vi "Find Resonances ASPT.vi"(8 "Error In":errorcluster, 11 "File Path Control":path=path "C:/Data/Spectra for Fedor/Ok spectra/300.00000K_175_555_2.10000V_0.00000T_May20-2015__09-37-18_001_052015.tdms") -> (0 "Error Out":errorcluster)   [LabVIEW 2016]
uses:
  Measure_extentions/Post-Processors/Line Detector/Line Detector Configuration.ctl
  <vilib>/Analysis/3filter.llb/Filter Passband Type.ctl
  <vilib>/Analysis/3filter.llb/Bessel Filter (CDB).vi
  Smooth Background CDBL.vi
  <vilib>/addons/Wavelet Analysis/application.llb/WA Multiscale Peak Detection (Array).vi
  <vilib>/Analysis/NI_AALPro.lvlib
  <vilib>/Analysis/NI_AAL_SigProc.lvlib
  <vilib>/Analysis/NI_AALBase.lvlib
  <vilib>/addons/_Advanced Signal Processing/NI_AdvSigProcWA.lvlib
panel:
  in  "ASPT?":bool
  out "# found":i32
  out "error":i32
  in  "Low pass distortion":dbl
  out "XY Graph 6":cluster{dbl[], dbl[]}[](graph)
  in  "User configuration":T1={"Peak width"=30.0} {"Peak width" format="%#_6pHz"}
  in  "Signal channel":string="Signal"
  in  "Frequency channel":string="Frequency"
  in  "group name in":string="p"
  in  "HP F":dbl=0.1 format="%#_6p"
  in  "LP  F":dbl=0.001 format="%#_6p"
  in  "Fit?":bool
  in  "Complex":bool
  in  "Deviations":dbl=1.0
  out "variance":dbl format="%.2p"
  out "standard deviation":dbl format="%.2p"
  out "Peak F":dbl format="%#_6pHz"
  in  "Points around peak":i32=100
  in  "Peak number":i32
  out "XY Graph 5":cluster{"Array":dbl[], "Array":dbl[]}[](graph)
  out "width":i32=100 min=3
  out "XY Graph 4":cluster{"Y":dbl[], dbl[]}(graph)
  out "XY Graph 3":cluster{"Y":dbl[], "Y":dbl[]}[](graph)
  out "Magnitude":cluster{"Y":dbl[], dbl[]}[](graph)
  out "Phase":cluster{"Y":dbl[], "Unwrapped Phase":dbl[]}[](graph)
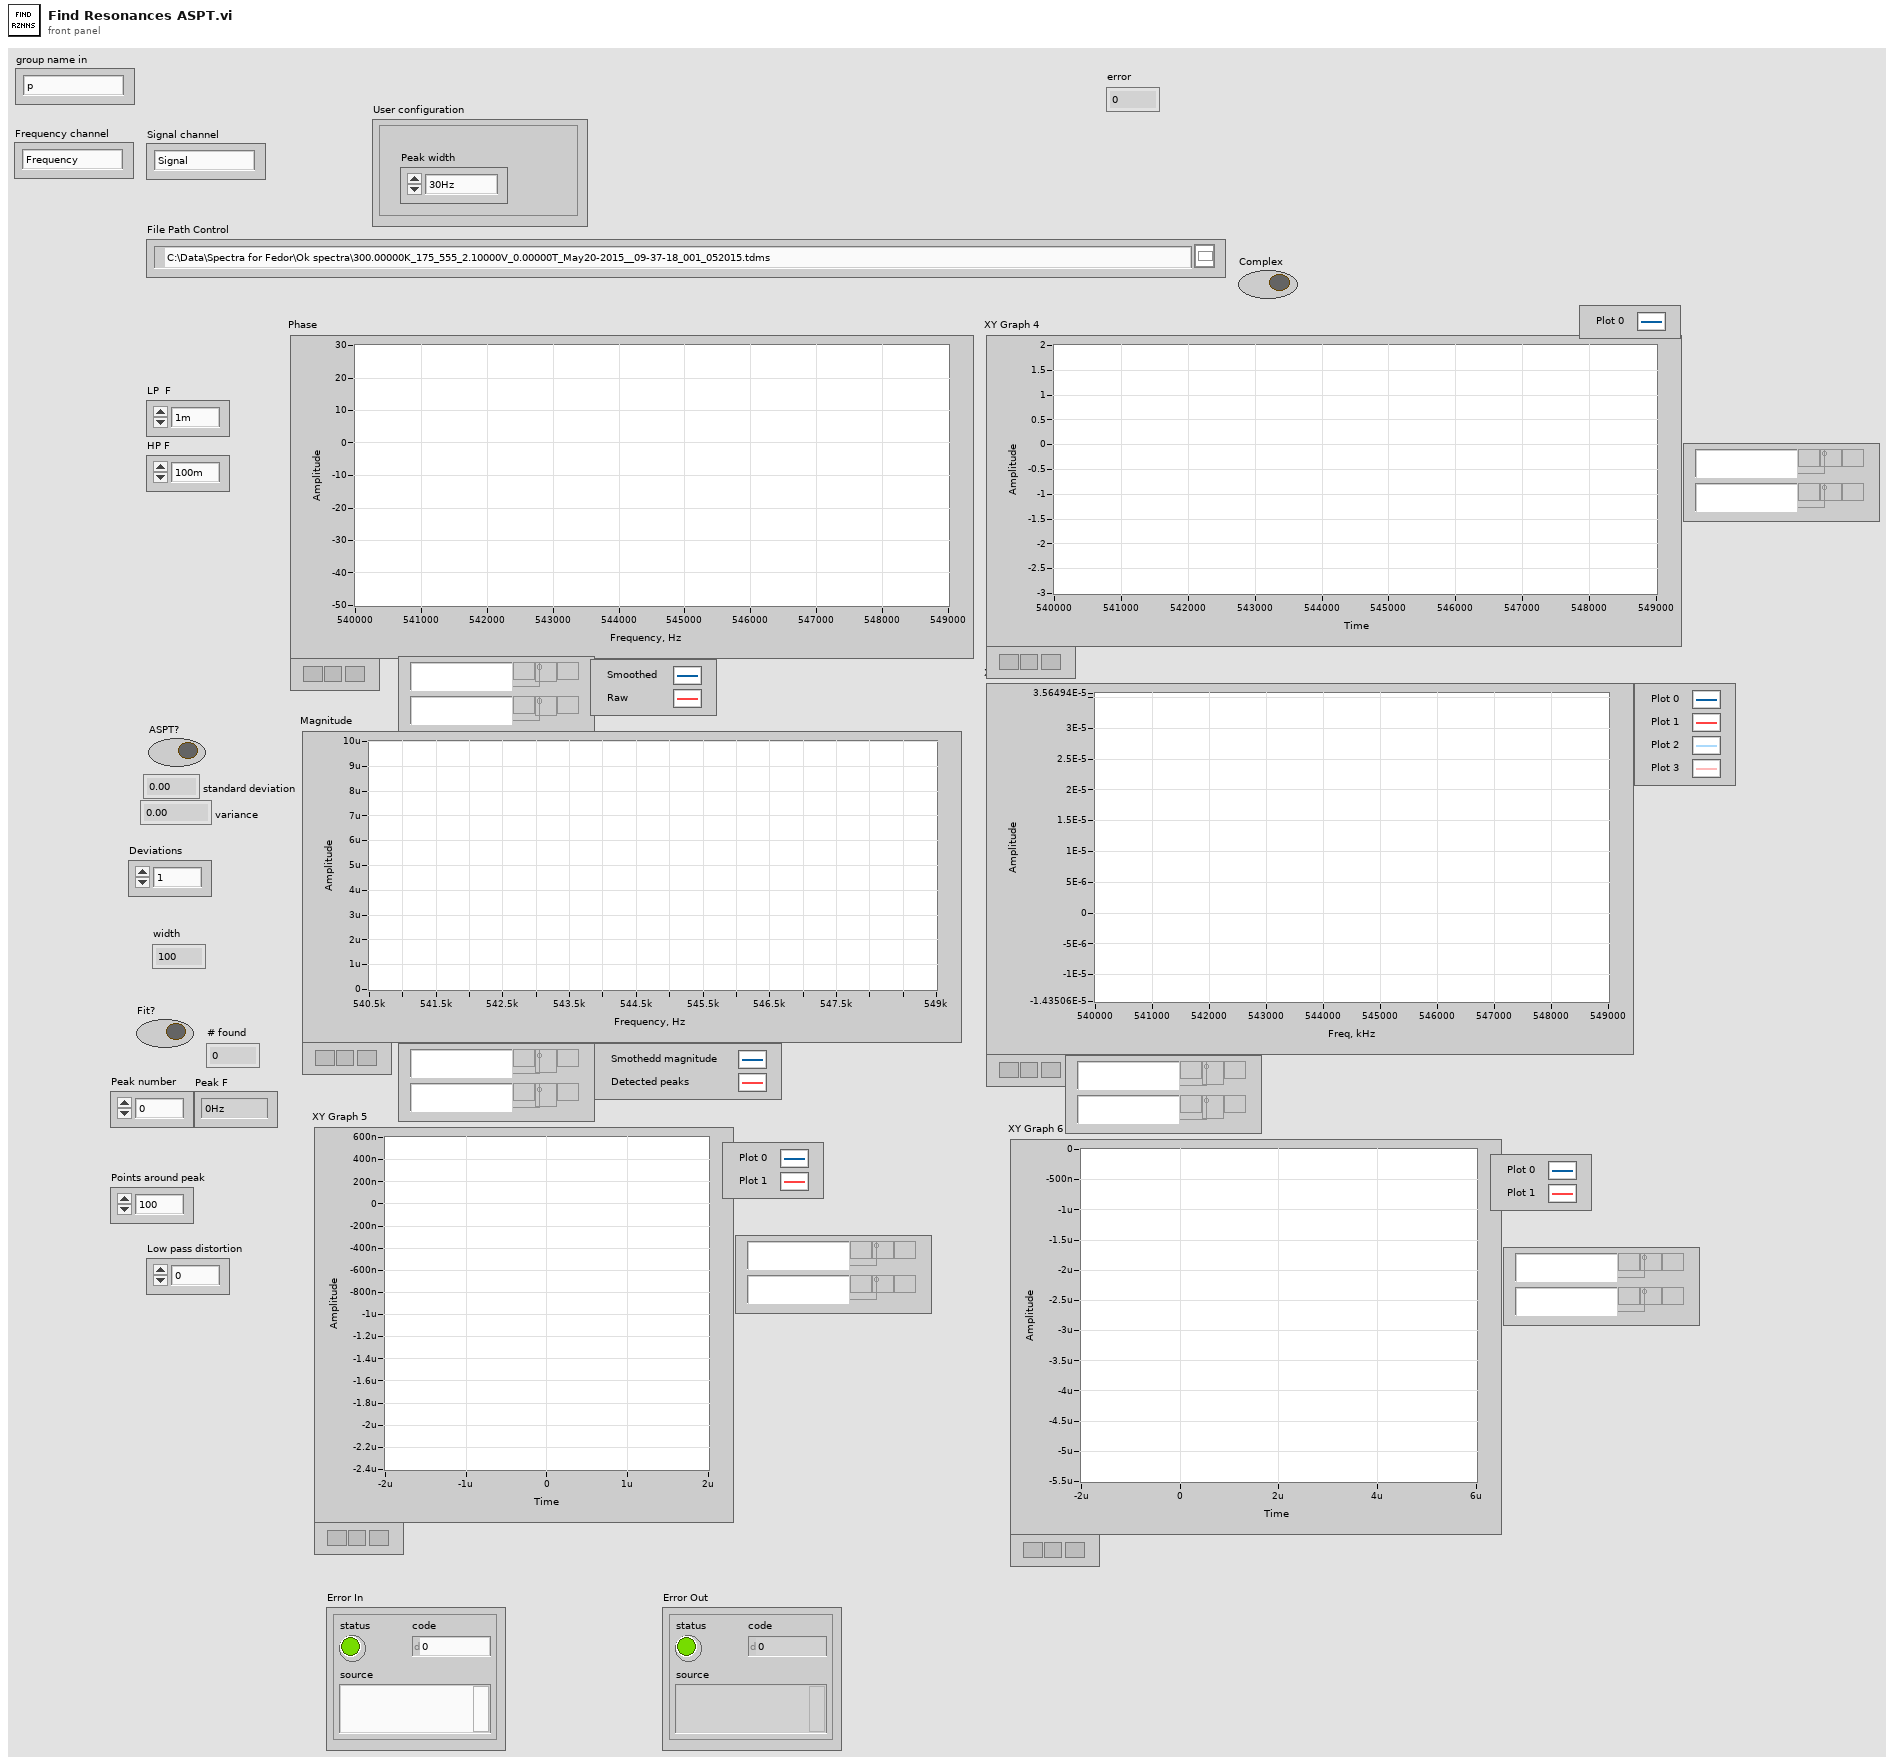
[diagram p1: front panel]
types:
  T1 = typedef "Line Detector Configuration.ctl" = cluster{"Peak width":dbl}
  T2 = enum16{"open", "open or create", "create or replace", "create", "open (read-only)"}
  T3 = typedef "NI_AALBase.lvlib/Filter Passband Type.ctl" = enum32{"Lowpass", "Highpass", "Bandpass", "Bandstop"}
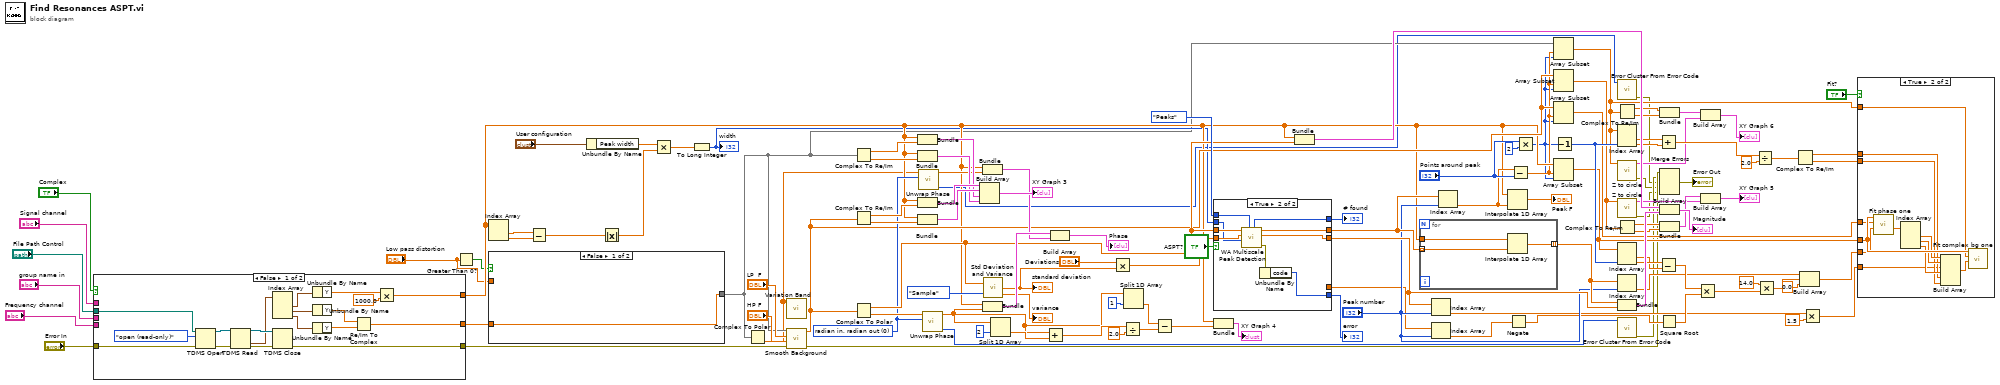
[diagram p0: block diagram]
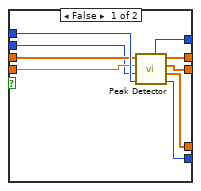
[diagram p2: hidden frame]
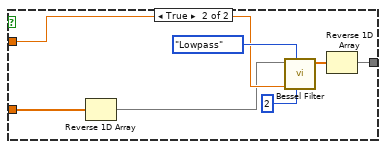
[diagram p3: hidden frame]
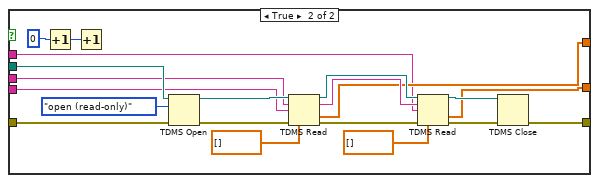
[diagram p5: hidden frame]
diagram:
  w81 = 0 items=["radian in, radian out", "radian in, degree out", "degree in, degree out", "degree in, radian out"] ("phase unit")
  n1 = case shown="False" "Complex" {
    tunnel: "File Path Control" -> [w137 w157]
    tunnel: [w121 w141] -> w40
    tunnel: "group name in" -> [_ w146]
    tunnel: "Frequency channel" -> [_ w145]
    tunnel: [w124 w142] -> w14
    tunnel: "Signal channel" -> [_ w140]
    tunnel: "Error In" -> [w123 w139]
    tunnel: [w122 w138] -> w41
    frame False {
      n2 = TDMS Open(8:w123, 10:T2."open (read-only)" ("operation (0:open)"), 11:w137) -> (0:w134:errorcluster, 3:w135:refnum<k34>)  [unwired: 4 in]
      n3 = TDMS Read(0:w135, 11:w134) -> (4:w133:refnum<k34>, 10:w131:waveform(dbl)[], 15:w132:errorcluster)  [unwired: 6 in, 3 out]
      n4 = Index Array(array=w131) -> (element #1=w130:waveform(dbl), element #2=w128:waveform(dbl), element #3=w129:waveform(dbl))  [unwired: 3 in]
      n5 = TDMS Close(8:w132, 11:w133) -> (0:w122:errorcluster)  [unwired: 1 out]
      n6 = Unbundle By Name(w130) -> ("Y"=w127:dbl[])
      n7 = Unbundle By Name(w128) -> ("Y"=w126:dbl[])
      n8 = Unbundle By Name(w129) -> ("Y"=w125:dbl[])
      n9 = Re/Im To Complex(1:w125, 2:w126) -> (0:w124:cdb[])
      n10 = Multiply(x=w127, y=1000.0) -> (x*y=w121:dbl[])
    }
    frame True {
      n11 = Increment(x=0 ("index")) -> (x+1=w151:i32)
      n12 = Increment(x=w151) -> ()  [unwired: 1 out]
      n13 = TDMS Open(8:w139, 10:T2."open (read-only)" ("operation (0:open)"), 11:w157) -> (0:w154:errorcluster, 3:w155:refnum<k34>)  [unwired: 4 in]
      n14 = TDMS Read(0:w155, 5:w146, 7:w145, 11:w154, 12:dbl[] []) -> (4:w149:refnum<k34>, 6:w147:string, 10:w141:dbl[], 15:w153:errorcluster)  [unwired: 3 in, 2 out]
      n15 = TDMS Read(0:w149, 5:w147, 7:w140, 11:w153, 12:cdb[] []) -> (4:w148:refnum<k34>, 10:w142:cdb[], 15:w150:errorcluster)  [unwired: 3 in, 3 out]
      n16 = TDMS Close(8:w150, 11:w148) -> (0:w138:errorcluster)  [unwired: 1 out]
    }
  }
  n17 = Greater Than 0?(x="Low pass distortion") -> (x > 0?=w16:bool)
  n18 = Index Array(array=w40) -> (element #1=w39:dbl, element #2=w38:dbl)  [unwired: 2 in]
  n19 = case shown="False" w16 {
    tunnel: w14 -> [w158 w165]
    tunnel: [w158 w159] -> w13
    tunnel: "Low pass distortion" -> [_ w162]
    frame False {
    }
    frame True {
      n20 = Reverse 1D Array(array=w165) -> (reversed array=w160:cdb[])
      n21 = call-poly <vilib>:"Bessel Filter.vi"("order"=2, "filter type"=Filter_Passband_Type."Lowpass", "low cutoff freq: fl"=w162, "X"=w160) -> ("Filtered X"=w164:cdb[])  [unwired: 4 in, 1 out]
      n22 = Reverse 1D Array(array=w164) -> (reversed array=w159:cdb[])
    }
  }
  n23 = Subtract(x=w39, y=w38) -> (x-y=w37:dbl)
  n24 = Unbundle By Name("User configuration") -> ("Peak width"=w35:dbl)
  n25 = Absolute Value(x=w37) -> (abs(x)=w34:dbl)
  n26 = Multiply(x=w35, y=w34) -> (x*y=w33:dbl)
  n27 = To Long Integer(number=w33) -> (32bit integer=w32:i32)
  "width" <- w32
  n28 = Complex To Polar(r * e^(i*theta)=w13) -> (theta=w2:dbl[])  [unwired: 1 out]
  n29 = call "Variation Band.vi"("Data"=w2) -> ()  [unwired: 11 in]
  n30 = call-poly "Smooth Background.vi"("Error In"=w41, "HP F"="HP F", "LP  F"="LP  F", "Data"=w13) -> ("Error Out"=w12:errorcluster, "Data out"=w52:cdb[])  [unwired: 6 in]
  n31 = Complex To Re/Im(x + iy=w13) -> (x=w91:dbl[], y=w92:dbl[])
  n32 = Complex To Re/Im(x + iy=w52) -> (x=w103:dbl[], y=w102:dbl[])
  n33 = Complex To Polar(r * e^(i*theta)=w52) -> (r=w88:dbl[], theta=w109:dbl[])
  n34 = Bundle(w40, w91) -> (w90:cluster{dbl[], dbl[]})  [unwired: 1 in]
  n35 = Bundle(w40, w92) -> (w89:cluster{dbl[], dbl[]})  [unwired: 1 in]
  n36 = Bundle(w40, w103) -> (w117:cluster{dbl[], dbl[]})  [unwired: 1 in]
  n37 = Bundle(w40, w102) -> (w116:cluster{dbl[], dbl[]})  [unwired: 1 in]
  n38 = call <vilib>:"Unwrap Phase.vi"("phase unit"=w81, "Phase"=w2) -> ("error"=w10:i32, "Unwrapped Phase"=w80:dbl[])  [unwired: 8 in]
  n39 = call <vilib>:"Unwrap Phase.vi"("phase unit"=w81, "Phase"=w109) -> ("error"=w11:i32, "Unwrapped Phase"=w104:dbl[])  [unwired: 8 in]
  n40 = Build Array(w117, w116, w90, w89) -> (→"XY Graph 3":cluster{dbl[], dbl[]}[])
  n41 = Bundle(w40, "Unwrapped Phase"=w80) -> (w78:cluster{dbl[], "Unwrapped Phase":dbl[]})  [unwired: 1 in]
  n42 = Bundle(w40, "Unwrapped Phase"=w104) -> (w118:cluster{dbl[], "Unwrapped Phase":dbl[]})  [unwired: 1 in]
  n43 = call <vilib>:"Std Deviation and Variance.vi"("X"=w88, "Weighting (Sample)"=enum16{"Sample", "Population"}."Sample") -> ("standard deviation"=w83:dbl, "variance"=→"variance":dbl)  [unwired: 1 out]
  "standard deviation" <- w83
  n44 = Split 1D Array(array=w104, index=2) -> (second subarray=w112:dbl[])  [unwired: 1 out]
  n45 = Add(x=w104, y=w112) -> (x+y=w111:dbl[])
  n46 = Build Array(w118, w78) -> (→"Phase":cluster{dbl[], "Unwrapped Phase":dbl[]}[])
  n47 = Multiply(x="Deviations", y=w83) -> (x*y=w84:dbl)
  n48 = Divide(x=w111, y=2.0) -> (x/y=w108:dbl[])
  n49 = Split 1D Array(array=w104, index=1) -> (second subarray=w105:dbl[])  [unwired: 1 out]
  n50 = Subtract(x=w105, y=w108) -> (x-y=w107:dbl[])
  n51 = case shown="True" "ASPT?" {
    tunnel: enum32{"Peaks", "Valleys"}."Peaks" ("peaks/valleys") -> [w174 w180]
    tunnel: w88 -> [w173 w183]
    tunnel: w84 -> [w172 w182]
    tunnel: [w171 w177] -> w75
    tunnel: [w170 w178] -> w70
    tunnel: [w169 _] -> w68
    tunnel: w32 -> [w168 w181]
    tunnel: [w167 w175] -> w4
    tunnel: [w166 w179] -> w3
    frame False {
      n52 = call <vilib>:"Peak Detector.vi"("peaks/valleys"=w174, "width"=w168, "threshold"=w172, "X"=w173) -> ("error"=w167:i32, "2nd Derivatives"=w169:dbl[], "Amplitudes"=w171:dbl[], "Locations"=w170:dbl[], "# found"=w166:i32)  [unwired: 3 in]
    }
    frame True {
      n53 = call-poly <vilib>:"WA Multiscale Peak Detection.vi"("peaks/valleys"=w180, "width"=w181, "threshold"=w182, "signal"=w183) -> ("error out"=w176:errorcluster, "amplitude"=w177:dbl[], "location"=w178:dbl[], "number of peaks"=w179:i32)  [unwired: 3 in, 1 out]
      n54 = Unbundle By Name(w176) -> ("code"=w175:i32)
    }
  }
  "error" <- w4
  "# found" <- w3
  n55 = Bundle(w40, w107) -> (→"XY Graph 4":cluster{dbl[], dbl[]})  [unwired: 1 in]
  n56 = Bundle(w40, w88) -> (w101:cluster{dbl[], dbl[]})  [unwired: 1 in]
  n57 = for {
    tunnel: w40 -> [w186]
    tunnel: w70 -> [w185] mode=indexing
    tunnel: [w184] -> w74 mode=indexing
    n58 = Interpolate 1D Array(1:w185, 2:w186) -> (0:w184:dbl)
  }
  n59 = Index Array(array=w75, index="Peak number") -> (element=w47:dbl)
  n60 = Index Array(array=w68, index="Peak number") -> (element=w67:dbl)
  n61 = Index Array(array=w70, index="Peak number") -> (element=w76:dbl)
  n62 = Interpolate 1D Array(1:w76, 2:w40) -> (0:→"Peak F":dbl)
  n63 = Negate(x=w67) -> (-x=w64:dbl)
  n64 = Subtract(x=w76, y="Points around peak") -> (x-y=w29:dbl)
  n65 = Multiply(x="Points around peak", y=2) -> (x*y=w28:i32)
  n66 = Array Subset(array=w13, index=w29, length=w28) -> (w22:cdb[])
  n67 = Array Subset(array=w52, index=w29, length=w28) -> (w20:cdb[])
  n68 = Array Subset(array=w52, index=w29, length=w28) -> (w53:cdb[])
  n69 = Array Subset(array=w40, index=w29, length=w28) -> (w27:dbl[])
  n70 = Decrement(x=w28) -> (x-1=w73:i32)
  n71 = call <vilib>:"Error Cluster From Error Code.vi"("error code (0)"=w10) -> ("error out"=w7:errorcluster)  [unwired: 8 in]
  n72 = Index Array(array=w22, index #2=w73) -> (element #1=w63:cdb, element #2=w62:cdb)  [unwired: 1 in]
  n73 = call "Z to circle.vi"("Z"=w22) -> ("Error Out"=w6:errorcluster, "plot"=w21:cluster{"Array":dbl[], "Array":dbl[]})  [unwired: 6 in, 3 out]
  n74 = call "Z to circle.vi"("Z"=w20) -> ("Error Out"=w5:errorcluster, "plot"=w18:cluster{"Array":dbl[], "Array":dbl[]})  [unwired: 6 in, 3 out]
  n75 = Index Array(array=w27, index #2=w73) -> (element #1=w71:dbl, element #2=w72:dbl)  [unwired: 1 in]
  n76 = Index Array(array=w74, index="Peak number") -> (element=w60:dbl)
  n77 = Bundle(w74, "amplitude"=w75) -> (w98:cluster{dbl[], "amplitude":dbl[]})  [unwired: 1 in]
  n78 = call <vilib>:"Error Cluster From Error Code.vi"("error code (0)"=w11) -> ("error out"=w8:errorcluster)  [unwired: 8 in]
  n79 = Complex To Re/Im(x + iy=w22) -> (x=w25:dbl[], y=w24:dbl[])
  n80 = Complex To Re/Im(x + iy=w20) -> (x=w95:dbl[], y=w94:dbl[])
  n81 = Add(x=w63, y=w62) -> (x+y=w61:cdb)
  n82 = Subtract(x=w72, y=w71) -> (x-y=w65:dbl)
  n83 = Square Root(x=w64) -> (sqrt(x)=w66:dbl)
  n84 = Bundle(w25, w24) -> (w26:cluster{dbl[], dbl[]})  [unwired: 1 in]
  n85 = Merge Errors(w12, w8, w7, w6, w5) -> (→"Error Out":errorcluster)
  n86 = Build Array(w101, w98) -> (→"Magnitude":cluster{dbl[], "amplitude":dbl[]}[])
  n87 = Bundle(w95, w94) -> (w19:cluster{dbl[], dbl[]})  [unwired: 1 in]
  n88 = Multiply(x=w65, y=w66) -> (x*y=w59:dbl)
  n89 = Build Array(w26, w21) -> (→"XY Graph 6":cluster{"Array":dbl[], "Array":dbl[]}[])
  n90 = Build Array(w19, w18) -> (→"XY Graph 5":cluster{"Array":dbl[], "Array":dbl[]}[])
  n91 = Divide(x=w61, y=2.0) -> (x/y=w56:cdb)
  n92 = Multiply(x=14.0, y=w59) -> (x*y=w31:dbl)
  n93 = Complex To Re/Im(x + iy=w56) -> (x=w55:dbl, y=w54:dbl)
  n94 = Build Array(w60, w31, 0.0 ("element")) -> (w57:dbl[])
  n95 = Multiply(x=w47, y=1.5) -> (x*y=w46:dbl)
  n96 = case shown="True" "Fit?" {
    tunnel: w22 -> [_ w197]
    tunnel: w27 -> [_ w198]
    tunnel: w57 -> [_ w196]
    tunnel: w46 -> [_ w188]
    tunnel: w55 -> [_ w191]
    tunnel: w54 -> [_ w190]
    tunnel: w53 -> [_ w187]
    frame False {
    }
    frame True {
      n97 = call "Fit phase one.vi"("Initial parameters"=w196, "Z"=w187, "X"=w198) -> ("best fit parameters"=w195:dbl[])  [unwired: 7 in, 1 out]
      n98 = Index Array(array=w195) -> (element #1=w194:dbl, element #2=w193:dbl, element #3=w192:dbl)  [unwired: 3 in]
      n99 = Build Array(w194, w193, w188, w192, w191, w190) -> (w189:dbl[])
      n100 = call "Fit complex bg one.vi"("Initial parameters"=w189, "Z"=w197, "X"=w198) -> ()  [unwired: 8 in, 1 out]
    }
  }
